vi "Seven Segment Decoder.vi"() -> ()   [LabVIEW 2015]
panel:
  out "e":bool
  out "d":bool
  out "c":bool
  out "f":bool
  out "b":bool
  out "g":bool
  out "a":bool
  in  "Boolean 4":bool
  in  "Boolean 3":bool
  in  "Boolean 2":bool
  in  "Boolean":bool
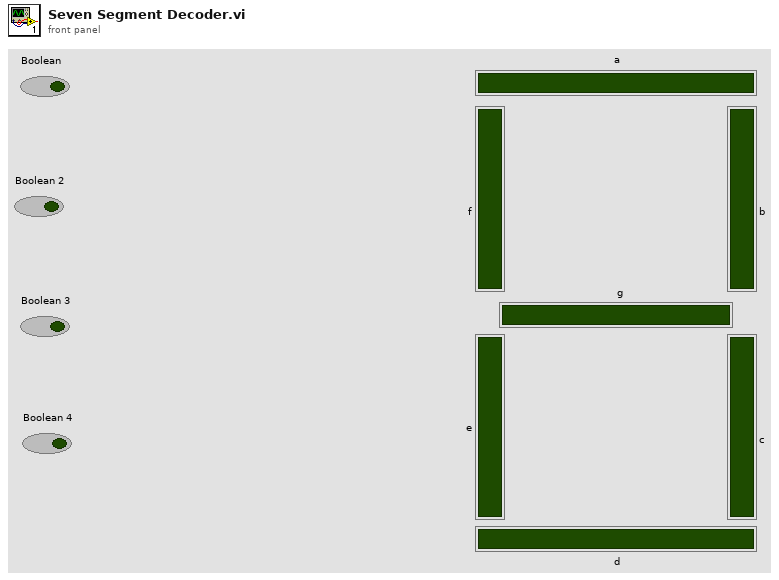
[diagram p1: front panel]
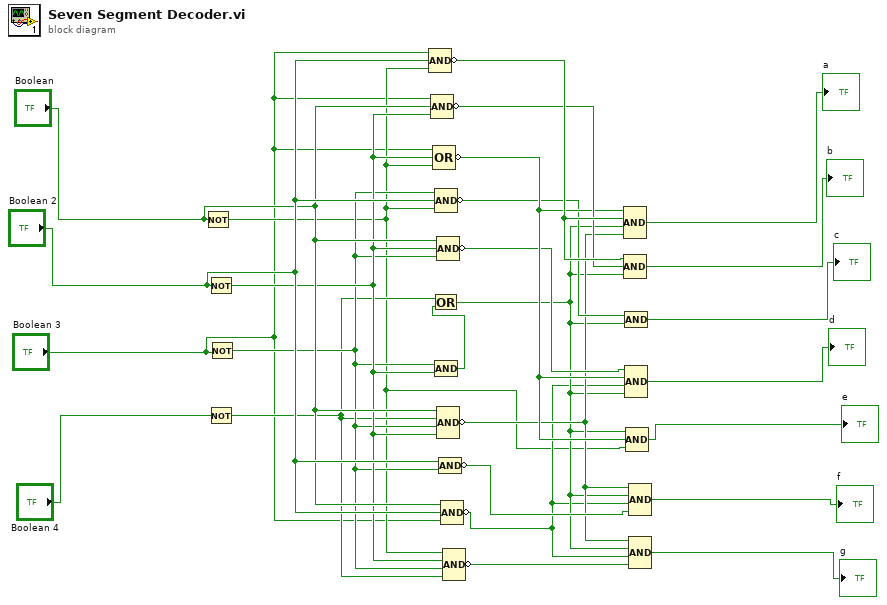
[diagram p0: block diagram]
diagram:
  n1 = Not(x="Boolean") -> (.not. x?=w9:bool)
  n2 = Not(x="Boolean 2") -> (.not. x?=w23:bool)
  n3 = Not(x="Boolean 4") -> (.not. x?=w21:bool)
  n4 = Not(x="Boolean 3") -> (.not. x?=w22:bool)
  n5 = Compound Arithmetic op=AND("Boolean 3", "Boolean 2", w9) -> (invert w19:bool)
  n6 = Compound Arithmetic op=AND("Boolean 3", "Boolean", w23) -> (invert w18:bool)
  n7 = Compound Arithmetic op=OR("Boolean 3", w23, w9) -> (invert w17:bool)
  n8 = Compound Arithmetic op=AND(w22, "Boolean 2", w9) -> (invert w16:bool)
  n9 = Compound Arithmetic op=AND(w22, w23) -> (w20:bool)
  n10 = Or(x=w21, y=w20) -> (x .or. y?=w11:bool)
  n11 = Compound Arithmetic op=AND("Boolean", w23, w22) -> (invert w15:bool)
  n12 = Compound Arithmetic op=AND("Boolean", w21, w22, w23) -> (invert w12:bool)
  n13 = Compound Arithmetic op=AND("Boolean 2", w22) -> (invert w13:bool)
  n14 = Compound Arithmetic op=AND("Boolean", "Boolean 2", "Boolean 3") -> (invert w10:bool)
  n15 = Compound Arithmetic op=AND(w9, w23, w22, w21) -> (invert w14:bool)
  n16 = Compound Arithmetic op=AND(w17, w19, w11, w12) -> (→"a":bool)
  n17 = Compound Arithmetic op=AND(w19, w18, w11) -> (→"b":bool)
  n18 = Compound Arithmetic op=AND(w16, w11) -> (→"c":bool)
  n19 = Compound Arithmetic op=AND(w15, w17, w10, w11) -> (→"d":bool)
  n20 = Compound Arithmetic op=AND(w11, w17, w9) -> (→"e":bool)
  n21 = Compound Arithmetic op=AND(w12, w11, w10, w13) -> (→"f":bool)
  n22 = Compound Arithmetic op=AND(w12, w11, w10, w14) -> (→"g":bool)
